vi "timeStamp_get.vi"(0 "TIME STRING IN":string, 2 "OPERATION":enum32{"Item 0", "Item 1"}(radio), 3 "TIME FORMAT":u16(ring) items=["MMM DD, YYYY", "YYMMDDhhmmss", "DD/MM/YY", "HH:MM:SS", "MMM DD, YYYY | hh:mm:ss,sss"]) -> (5 "TIME STRING OUT":string, 6 "TIME STAMP OUT":timestamp format="%<%x %.3X>T", 7 "SUCCESS?":bool)   [LabVIEW 2018, in "db_lib R3.lvlib"]
uses:
  db_lib R3.lvlib
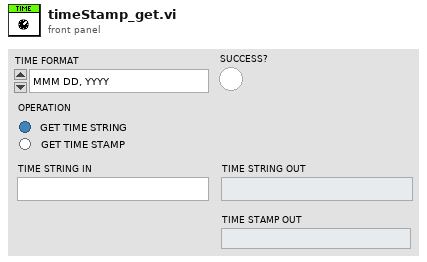
[diagram p1: front panel]
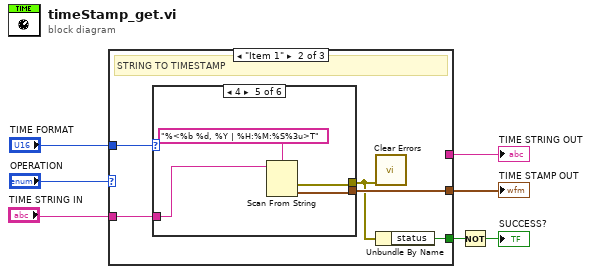
[diagram p0: block diagram]
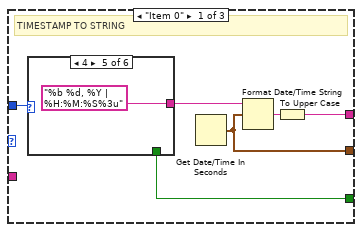
[diagram p2: hidden frame]
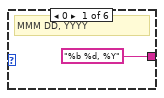
[diagram p3: hidden frame]
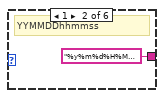
[diagram p4: hidden frame]
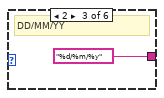
[diagram p5: hidden frame]
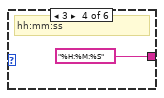
[diagram p6: hidden frame]
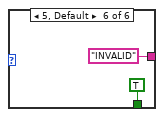
[diagram p7: hidden frame]
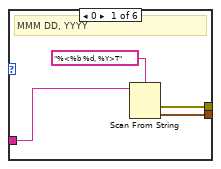
[diagram p8: hidden frame]
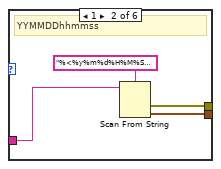
[diagram p9: hidden frame]
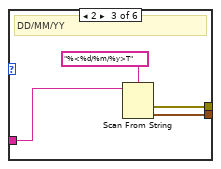
[diagram p10: hidden frame]
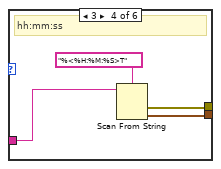
[diagram p11: hidden frame]
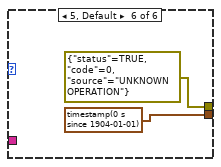
[diagram p12: hidden frame]
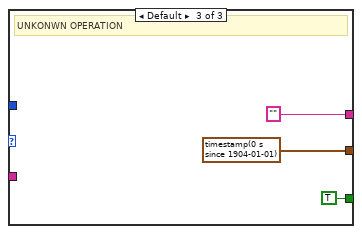
[diagram p13: hidden frame]
diagram:
  n1 = case shown="\"Item 1\"" "OPERATION" {
    tunnel: "TIME FORMAT" -> [w13 w25 _]
    tunnel: [w10 _ ""] -> w5
    tunnel: [w9 w24 timestamp(0 s since 1904-01-01)] -> w4
    tunnel: "TIME STRING IN" -> [_ w23 _]
    tunnel: [w8 w21 TRUE ("status")] -> w2
    frame "Item 0" {
      # "TIMESTAMP TO STRING"
      n2 = case shown="4" w13 {
        tunnel: ["%b %d, %Y" "%y%m%d%H%M%S" "%d/%m/%y" "%H:%M:%S" "%b %d, %Y | %H:%M:%S%3u" "INVALID"] -> w12
        tunnel: [_ _ _ _ _ TRUE] -> w8
        frame 0 {
          # "MMM DD, YYYY"
        }
        frame 1 {
          # "YYMMDDhhmmss"
        }
        frame 2 {
          # "DD/MM/YY"
        }
        frame 3 {
          # "hh:mm:ss"
        }
        frame 4 {
        }
        frame 5, Default {
        }
      }
      n3 = Get Date/Time In Seconds() -> (seconds since 1Jan1904=w9:timestamp)
      n4 = Format Date/Time String(time format string (%c)=w12, seconds (now)=w9) -> (date/time string=w11:string)  [unwired: 1 in]
      n5 = To Upper Case(1:w11) -> (0:w10:string)
    }
    frame "Item 1" {
      # "STRING TO TIMESTAMP"
      n6 = case shown="4" w25 {
        tunnel: [w28 w32 w36 w40 w42 timestamp(0 s since 1904-01-01)] -> w24
        tunnel: w23 -> [w27 w31 w35 w39 w44 _]
        tunnel: [w26 w30 w34 w38 w43 errorcluster {"status"=TRUE, "code"=0, "source"="UNKNOWN OPERATION"} ("error IO")] -> w22
        frame 0 {
          # "MMM DD, YYYY"
          n7 = Scan From String(format string="%<%b %d, %Y>T", input string=w27) -> (error out=w26:errorcluster, output 1=w28:timestamp)  [unwired: 3 in, 2 out]
        }
        frame 1 {
          # "YYMMDDhhmmss"
          n8 = Scan From String(format string="%<%y%m%d%H%M%S>T", input string=w31) -> (error out=w30:errorcluster, output 1=w32:timestamp)  [unwired: 3 in, 2 out]
        }
        frame 2 {
          # "DD/MM/YY"
          n9 = Scan From String(format string="%<%d/%m/%y>T", input string=w35) -> (error out=w34:errorcluster, output 1=w36:timestamp)  [unwired: 3 in, 2 out]
        }
        frame 3 {
          # "hh:mm:ss"
          n10 = Scan From String(format string="%<%H:%M:%S>T", input string=w39) -> (error out=w38:errorcluster, output 1=w40:timestamp)  [unwired: 3 in, 2 out]
        }
        frame 4 {
          n11 = Scan From String(format string="%<%b %d, %Y | %H:%M:%S%3u>T", input string=w44) -> (error out=w43:errorcluster, output 1=w42:timestamp)  [unwired: 3 in, 2 out]
        }
        frame 5, Default {
        }
      }
      n12 = call <vilib>:"Clear Errors.vi"("error in (no error)"=w22) -> ()  [unwired: 5 in, 2 out]
      n13 = Unbundle By Name(w22) -> ("status"=w21:bool)
    }
    frame Default {
      # "UNKONWN OPERATION"
    }
  }
  "TIME STAMP OUT" <- w4
  "TIME STRING OUT" <- w5
  n14 = Not(x=w2) -> (.not. x?=→"SUCCESS?":bool)
